vi "gas.vi"(10 "Slide":u8(slide) scale=0.0..12.0, 11 "Array":T1[](array[typedef]) {"Data" format="%.0x"}) -> (3 "Array 2":T1[](array[typedef]) {"Data" format="%.0x"})   [LabVIEW 2021, in "uCanDriver.lvlib" / "uCAN.lvclass"]
uses:
  uCAN.lvclass
  typedefs/frame.ctl
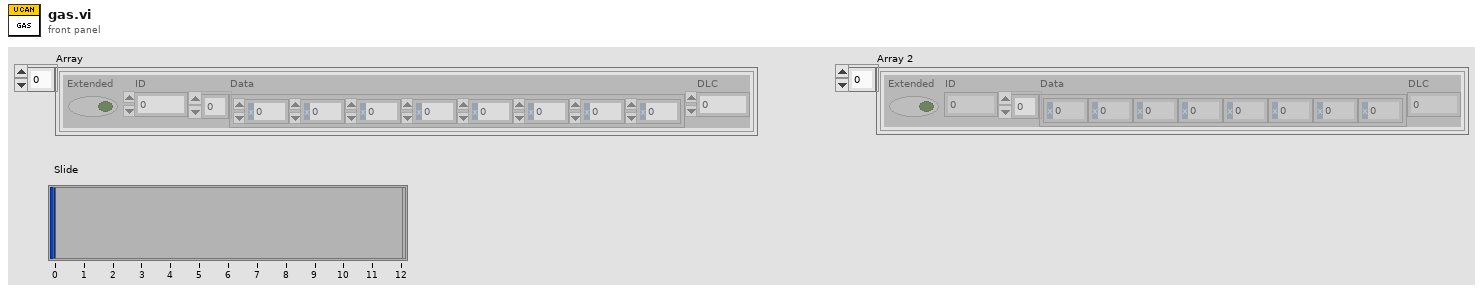
[diagram p1: front panel]
types:
  T1 = typedef "uCanDriver.lvlib/uCAN.lvclass/frame.ctl" = cluster{"Extended":bool, "ID":u32, "Data":u8[], "DLC":u8}
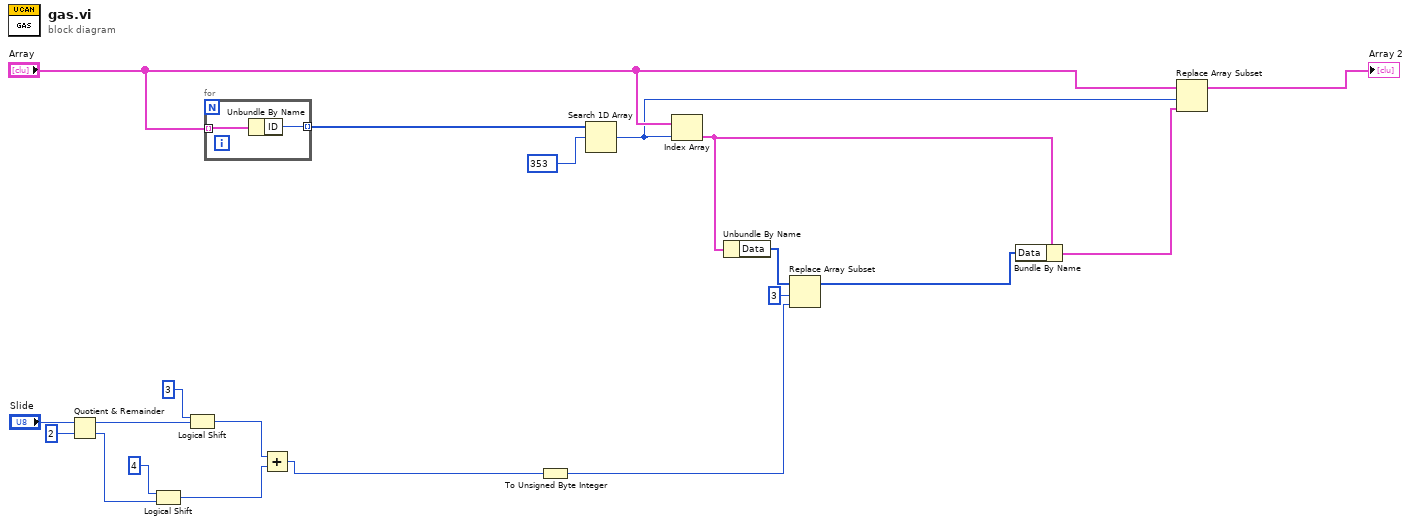
[diagram p0: block diagram]
diagram:
  n1 = Quotient & Remainder(x="Slide", y=u8 2) -> (x-y*floor(x/y)=w4:u8, floor(x/y)=w5:u8)
  n2 = Logical Shift(y=i16 4, x=w5) -> (x << y=w2:u8)
  n3 = Logical Shift(y=i16 3, x=w4) -> (x << y=w3:u8)
  n4 = for {
    tunnel: "Array" -> [w22] mode=indexing
    tunnel: [w21] -> w18 mode=indexing
    n5 = Unbundle By Name(w22) -> ("ID"=w21:u32)
  }
  n6 = Add(x=w3, y=w2) -> (x+y=w1:u8)
  n7 = To Unsigned Byte Integer(number=w1) -> (unsigned 8bit integer=w10:u8)
  n8 = Search 1D Array(1D array=w18, element=u32 353) -> (index of element=w16:i32)  [unwired: 1 in]
  n9 = Index Array(array="Array", index=w16) -> (element=w20:T1)
  n10 = Unbundle By Name(w20) -> ("Data"=w13:u8[])
  n11 = Replace Array Subset(array=w13, new element=w10, index=3) -> (w11:u8[])
  n12 = Bundle By Name(cluster=w20, "Data"=w11) -> (w14:T1)
  n13 = Replace Array Subset(array="Array", new element=w14, index=w16) -> (→"Array 2":T1[])
